vi "AMI_SetCampo XYZ axis.vi"(6 "error in (no error)":errorcluster, 7 "Index":i8) -> (0 "error out":errorcluster, 3 "resulting string Z":string="Set Magnetic Field 1000.000Tesla at 100.000Tesla/min, Linear, Persistent, Sweep&meas")   [LabVIEW 2017]
doc: "Use this template to create a dialog box. This template polls the state of the buttons on the front panel and does not use events. Use the Dialog Using Events template (not available in Base package) to create a dialog box with event handling."
panel:
  in  "Measure cDAQ":bool=TRUE
  in  "Y factor":dbl=0.03 min=0.0 max=0.1 step=0.001 format="%.3f"
  in  "X factor":dbl=0.03 min=0.0 max=0.1 step=0.001 format="%.3f"
  in  "Modo Rampa":u16(ring) items=["RAMP", "PAUSE", "MANUAL UP", "MANUAL DOWN", "ZERO"]
  out "Z Ramp Units":u16(ring)=1 items=["Per SECOND", "Per MINUTE"]
  out "Z Field Units":u16(ring)=1 items=["KGauss", "Tesla"]
  out "Wait until stable":bool=TRUE
  in  "Field Mode":i32(ring) items=["Persistent", "Driven"]
  in  "Approach":i32(ring) items=["Linear", "NoOvershoot", "Oscillate"]
  in  "Z rate":dbl=0.03 min=0.0 max=0.1 step=0.001 format="%.3f"
  in  "Z target":dbl=0.1 min=-2.0 max=2.0 format="%.3f"
  out "Cancelled?":bool
  in  "Cancel":bool
  in  "OK":bool
  # "XYZ  MAGNETIC FIELD"
  # "Enero 2023 V2.1  a-sslcdms"
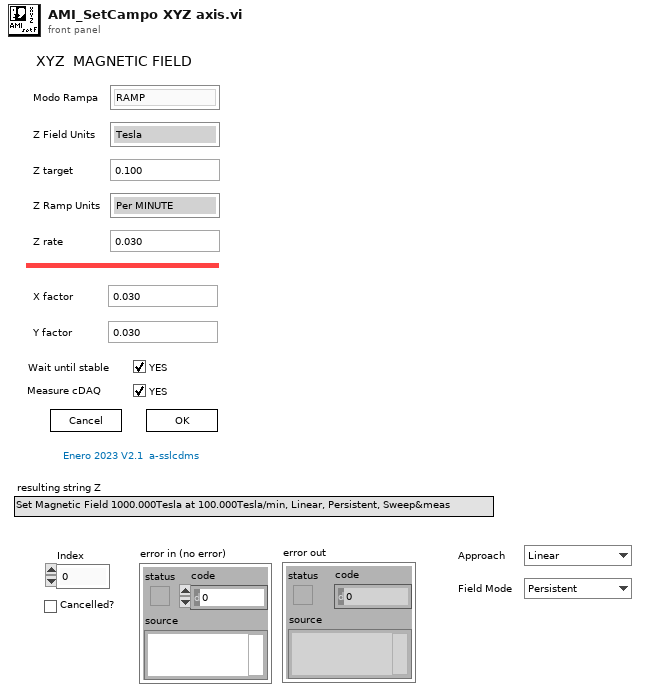
[diagram p1: front panel]
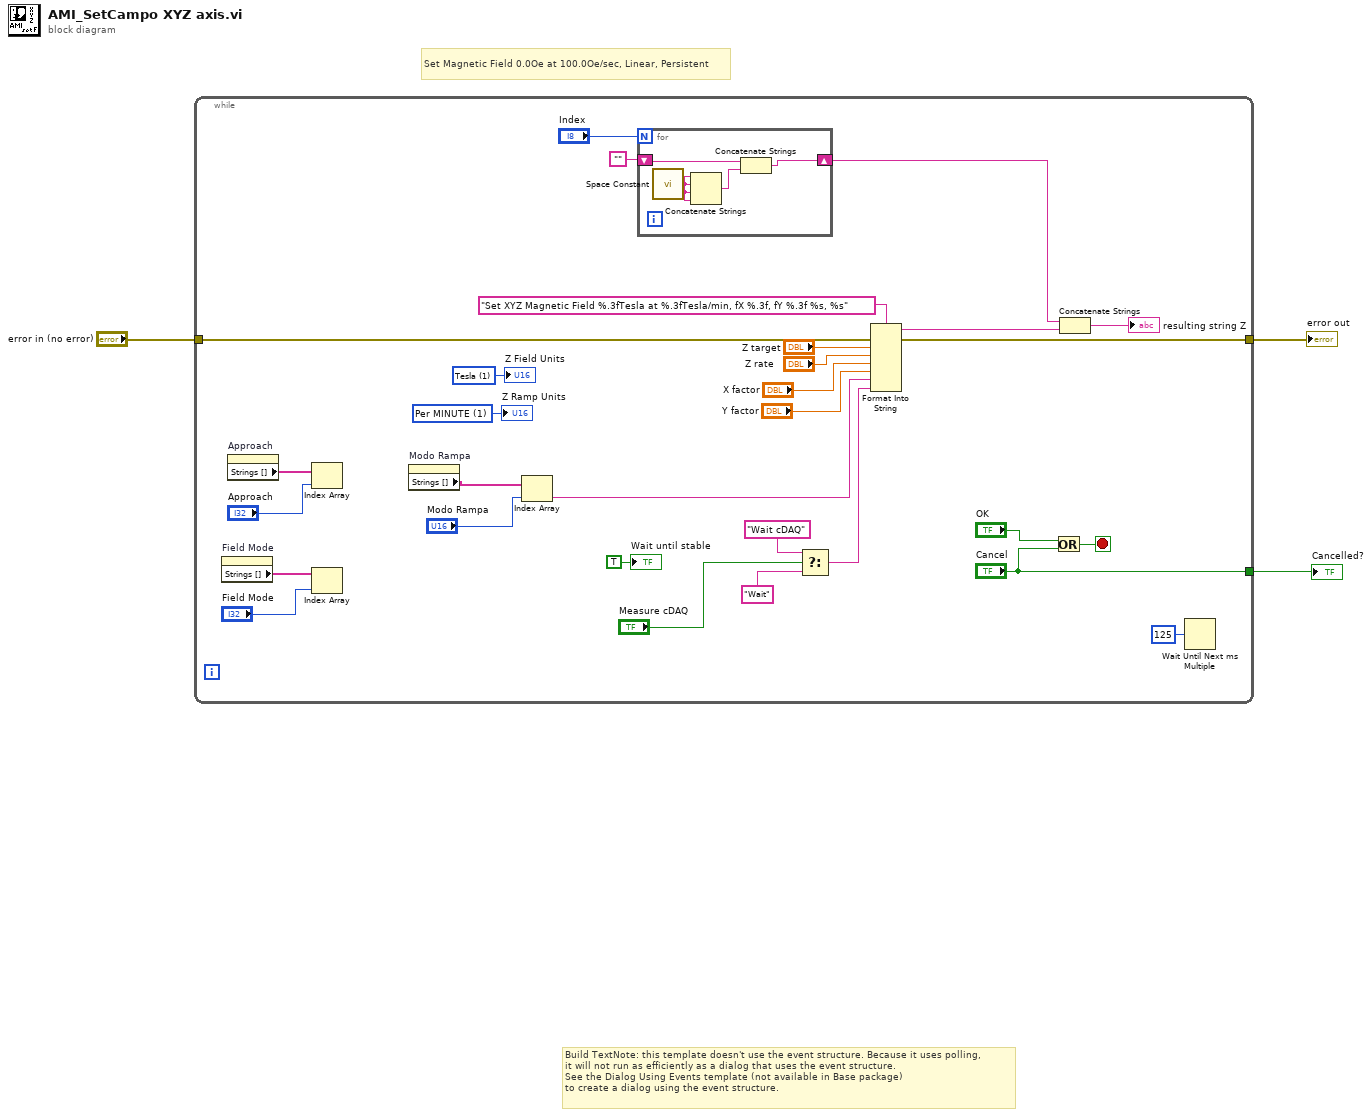
[diagram p0: block diagram]
diagram:
  # "Set Magnetic Field 0.0Oe at 100.0Oe/sec, Linear, Persistent"
  # "Build TextNote: this template doesn't use the event structure. Because it uses polling, \nit will not run as efficiently as a dialog that uses the event structure.\nSee the Dialog Using Events template (not available in Base package) \nto create a dialog using the event structure."
  n1 = while {
    tunnel: ["Cancel"] -> w3
    tunnel: [w11] -> w2
    tunnel: "error in (no error)" -> [w13]
    stop <- w32 stop-if-true
    w14 = u16 1 items=["Per SECOND", "Per MINUTE"] ("Ramp Units")
    w15 = u16 1 items=["KGauss", "Tesla"] ("Field Units")
    n2 = property on="Field Mode" class="Ring (strict)"() -> ("Strings []"=w21:string[])  [unwired: 2 in, 2 out]
    n3 = property on="Approach" class="Ring (strict)"() -> ("Strings []"=w24:string[])  [unwired: 2 in, 2 out]
    n4 = Index Array(array=w24, index="Approach") -> ()  [unwired: 1 out]
    n5 = Index Array(array=w21, index="Field Mode") -> ()  [unwired: 1 out]
    n6 = property on="Modo Rampa" class="Ring (strict)"() -> ("Strings []"=w9:string[])  [unwired: 2 in, 2 out]
    n7 = Index Array(array=w9, index="Modo Rampa") -> (element=w5:string)
    n8 = for {
      N: "Index" -> [_]
      shift-right: [w36] -> w12
      shift-left: "" -> [w35]
      n9 = call <vilib>:"Space Constant.vi"() -> ("String"=w34:string)
      n10 = Concatenate Strings(w34, w34, w34, w34) -> (w37:string)
      n11 = Concatenate Strings(w35, w37) -> (w36:string)
    }
    n12 = Select(t="Wait cDAQ", s="Measure cDAQ", f="Wait") -> (s? t:f=w8:string)
    n13 = Format Into String(format string="Set XYZ Magnetic Field %.3fTesla at %.3fTesla/min, fX %.3f, fY %.3f %s, %s", error in=w13, "Z target", "Z rate", "X factor", "Y factor", w5, w8) -> (resulting string=w26:string, error out=w11:errorcluster)  [unwired: 1 in]
    n14 = Or(x="OK", y="Cancel") -> (x .or. y?=w32:bool)
    n15 = Concatenate Strings(w12, w26) -> (→"resulting string Z":string)
    n16 = Wait Until Next ms Multiple(millisecond multiple=u32 125) -> ()  [unwired: 1 out]
    "Wait until stable" <- TRUE ("Wait stability")
    "Z Field Units" <- w15
    "Z Ramp Units" <- w14
  }
  "Cancelled?" <- w3
  "error out" <- w2
